vi "Measure Voltage.vi"(8 "error in":errorcluster, 11 "ManualPS in":refnum<class "ManualPS.lvclass">) -> (0 "error out":errorcluster, 2 "Voltage":dbl, 3 "ManualPS out":refnum<class "ManualPS.lvclass">)   [LabVIEW 2018, in "ManualPS.lvlib" / "ManualPS.lvclass"]
uses:
  ManualPS.lvclass
  builds/Power_Supply.lvlibp/Power Supply.lvclass
  C:/Users/Ron.Dexter.LUMINARTECH/Desktop/builds/Power_Supply.lvlibp/Power Supply.lvclass
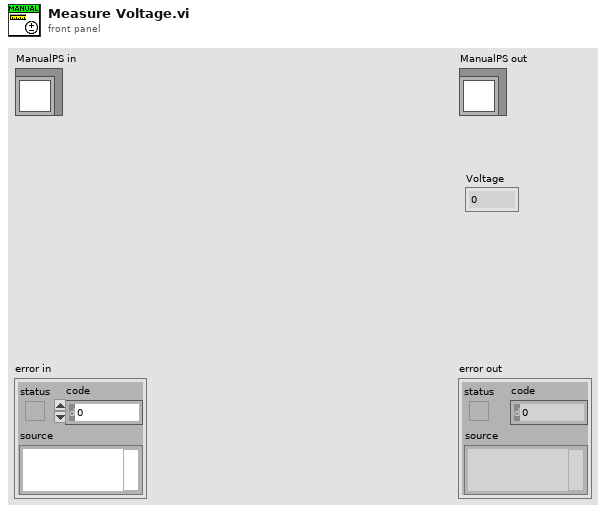
[diagram p1: front panel]
types:
  T1 = typedef "Power_Supply.lvlibp/Supply Settings.ctl" = cluster{"Voltage":dbl, "Current":dbl, "Output":bool}
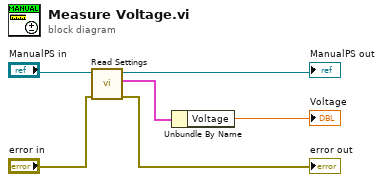
[diagram p0: block diagram]
diagram:
  n1 = call "Read Settings.vi"("error in (no error)"="error in", "Power Supply in"="ManualPS in") -> ("error out"=→"error out":errorcluster, "Settings"=w4:T1, "Power Supply out"=→"ManualPS out":refnum<class "ManualPS.lvclass">)  [unwired: 7 in]
  n2 = Unbundle By Name(w4) -> ("Voltage"=→"Voltage":dbl)
